vi "Transform48To48.vi"(8 "error in (no error)":errorcluster, 9 "Max Output Value":u16, 10 "Demosaicked Data":u16[](array[numeric]), 11 "ColorProcessor reference in":refnum<k24>) -> (0 "error out":errorcluster, 2 "outputData":u16[](array[numeric]), 3 "ColorProcessor reference out":refnum<k24>)   [LabVIEW 2022 SP3]
uses:
  I:/.shortcut-targets-by-id/1riZacJd_1_jmKfGgrjDuP7KcecvMS3i2/Xiao research group/Programs/XYZRecorrection/Scientific Camera Interfaces/SDK/DotNet Toolkit/dlls/Managed_64_lib/Thorlabs.TSI.ColorInterfaces.dll
  SDK/DotNet Toolkit/dlls/Managed_64_lib/Thorlabs.TSI.ColorInterfaces.dll
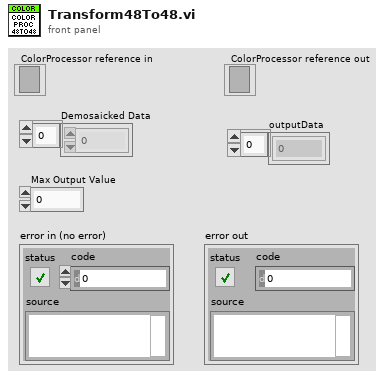
[diagram p1: front panel]
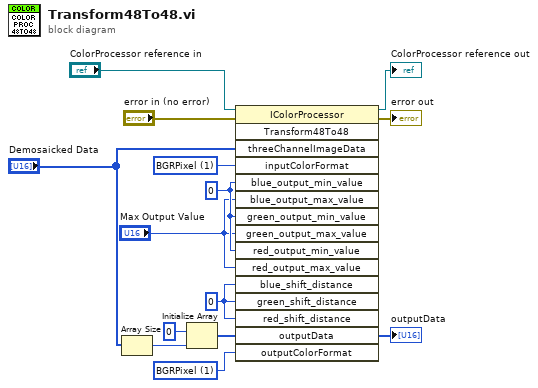
[diagram p0: block diagram]
diagram:
  w8 = 1 items=["BGRPlanar", "BGRPixel", "RGBPixel"] ("outputColorFormat")
  w7 = 0 ("blue_shift_distance")
  w6 = u16 0 ("blue_output_min_value")
  w4 = 1 items=["BGRPlanar", "BGRPixel", "RGBPixel"] ("inputColorFormat")
  n1 = Array Size(array="Demosaicked Data") -> (size(s)=w11:i32)
  n2 = Initialize Array(u16 0 ("element"), w11) -> (w12:u16[])
  n3 = invoke class="IColorProcessor" method="Transform48To48"(reference="ColorProcessor reference in", error in="error in (no error)", "threeChannelImageData"="Demosaicked Data", "inputColorFormat"=w4, "blue_output_min_value"=w6, "blue_output_max_value"="Max Output Value", "green_output_min_value"=w6, "green_output_max_value"="Max Output Value", "red_output_min_value"=w6, "red_output_max_value"="Max Output Value", "blue_shift_distance"=w7, "green_shift_distance"=w7, "red_shift_distance"=w7, "outputData"=w12, "outputColorFormat"=w8) -> (reference out=→"ColorProcessor reference out":refnum<k24>, error out=→"error out":errorcluster, "outputData"=→"outputData":u16[])  [unwired: 1 in, 13 out]
